vi "split by relative paths.vi"(10 "base path":path, 11 "paths to search":path[](array[path])) -> (1 "relative from path to base":path[](array[path]), 2 "relative":path[](array[path]), 3 "not relative":path[](array[path]))   [LabVIEW 2014]
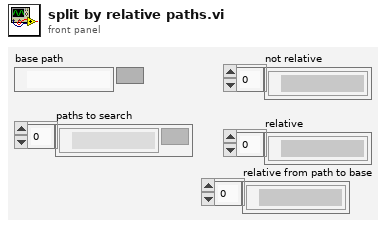
[diagram p1: front panel]
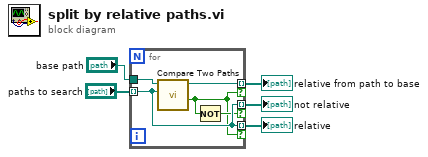
[diagram p0: block diagram]
diagram:
  n1 = for {
    tunnel: "paths to search" -> [w9] mode=indexing
    tunnel: "base path" -> [w10]
    tunnel: [w9] -> w4 mode=indexing if=w8
    tunnel: [w9] -> w5 mode=indexing if=w6
    tunnel: [w7] -> w1 mode=indexing if=w6
    n2 = call <vilib>:"Compare Two Paths.vi"("Path 2"=w9, "Path 1"=w10) -> ("Path 2 Relative to Path 1?"=w6:bool, "Relative Path from 1 to 2"=w7:path)  [unwired: 6 in, 2 out]
    n3 = Not(x=w6) -> (.not. x?=w8:bool)
  }
  "relative" <- w5
  "not relative" <- w4
  "relative from path to base" <- w1
